vi "Demodulator.vi"(5 "Initial df":dbl, 7 "rx":cdb[](array[numeric]), 9 "I":cdb[](array[numeric])) -> (8 "all symbols":cdb[][](array[numeric]))   [LabVIEW 2017]
uses:
  <vilib>/Analysis/2dsp.llb/Upsample (CDB).vi
  <vilib>/Analysis/3filter.llb/FIR Filter (CDB).vi
  <vilib>/Analysis/NI_AALBase.lvlib
  <vilib>/Analysis/NI_AALPro.lvlib
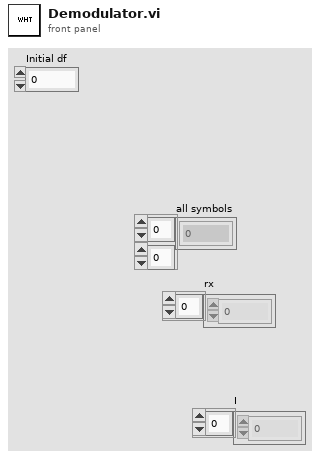
[diagram p1: front panel]
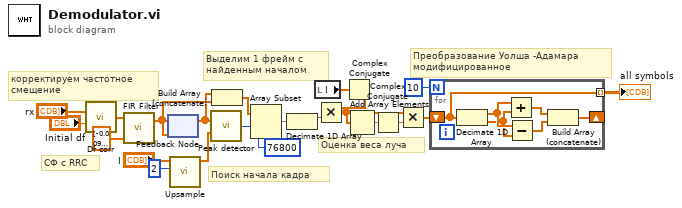
[diagram p0: block diagram]
diagram:
  # "Оценка веса луча"
  # "Поиск начала кадра"
  # "корректируем частотное \nсмещение"
  # "Выделим 1 фрейм с\nнайденным началом"
  # "СФ с RRC"
  # "Преобразование Уолша -Адамара\nмодифицированное"
  n1 = call "Df corr.vi"("in"="rx", "df"="Initial df") -> ("out"=w8:cdb[])  [unwired: 13 in]
  n2 = call-poly <vilib>:"FIR Filter.vi"("FIR Coefficients"=dbl[] [-0.00950243582382866, 0.0038289020696010124, 0.017986614233027234, -0.021118983745163862, -0.02699793163067473, 0.05461330061406498, 0.03500744412796962, -0.1267561574637285, -0.04053385271622267, 0.44202811643652723, 0.7496128788800704, 0.44202811643652723, -0.04053385271622267, -0.1267561574637285, 0.03500744412796962, 0.05461330061406498, -0.02699793163067473, -0.021118983745163862, 0.017986614233027234, 0.0038289020696010124, -0.00950243582382866] ("Дискретизированная импульсная характеристика(коэффициенты) 2"), "X"=w8) -> ("Filtered X"=w7:cdb[])  [unwired: 2 in, 1 out]
  n3 = feedback #1(w7) -> (w6:cdb[])
  n4 = feedback-in #1(w7) -> ()
  n5 = call-poly <vilib>:"Upsample.vi"("upsampling factor"=2, "X"="I") -> ("Upsampled Array"=w12:cdb[])  [unwired: 8 in, 1 out]
  n6 = call "Peak detector.vi"("X"=w6, "Y"=w12) -> ("peak\nindex"=w2:i32)  [unwired: 11 in, 2 out]
  n7 = Build Array (concatenate)(w6, w7) -> (w16:cdb[])
  n8 = Array Subset(array=w16, index=w2, length=76800) -> (w15:cdb[])
  n9 = Decimate 1D Array(w15) -> (w1:cdb[])  [unwired: 1 out]
  n10 = local read "I"() -> (w4:cdb[])
  n11 = Complex Conjugate(1:w4) -> (0:w3:cdb[])
  n12 = Multiply(x=w3, y=w1) -> (x*y=w21:cdb[])
  n13 = Add Array Elements(numeric array=w21) -> (sum=w18:cdb)
  n14 = Complex Conjugate(1:w18) -> (0:w19:cdb)
  n15 = Multiply(x=w21, y=w19) -> (x*y=w20:cdb[])
  n16 = for {
    N: 10 -> [_]
    shift-right: [w24] -> _
    shift-left: w20 -> [w23]
    tunnel: [w23] -> w17 mode=indexing
    n17 = Decimate 1D Array(w23) -> (w28:cdb[], w27:cdb[])
    n18 = Add(x=w28, y=w27) -> (x+y=w25:cdb[])
    n19 = Subtract(x=w28, y=w27) -> (x-y=w26:cdb[])
    n20 = Build Array (concatenate)(w25, w26) -> (w24:cdb[])
  }
  "all symbols" <- w17
